vi "Read gesture + average_speed + abs speed - Leap.vi"() -> ()   [LabVIEW 2014]
uses:
  <vilib>/Utility/file.llb/Write To Spreadsheet File (DBL).vi
panel:
  in  "Save":bool
  out "Average Speed":T1(graph)
  out "Absolute speed":T2(graph)
  in  "Acquire":bool
  out "Finger pinch":bool[](array[boolean])
  out "Key tap":string[](array[string])=["Undetected", "Undetected", "Undetected", "Undetected", "Undetected"]
  in  "Key Tap Thresh [degree]":sgl=55.0 caption="Keytap Threshold [degree]"
  out "Wrist Flexion/Extension":string="Undetected"
  in  "Flex-Extension Threshold [degree]":sgl=40.0
  out "Palm State":string="Undetected"
  in  "Stop":bool
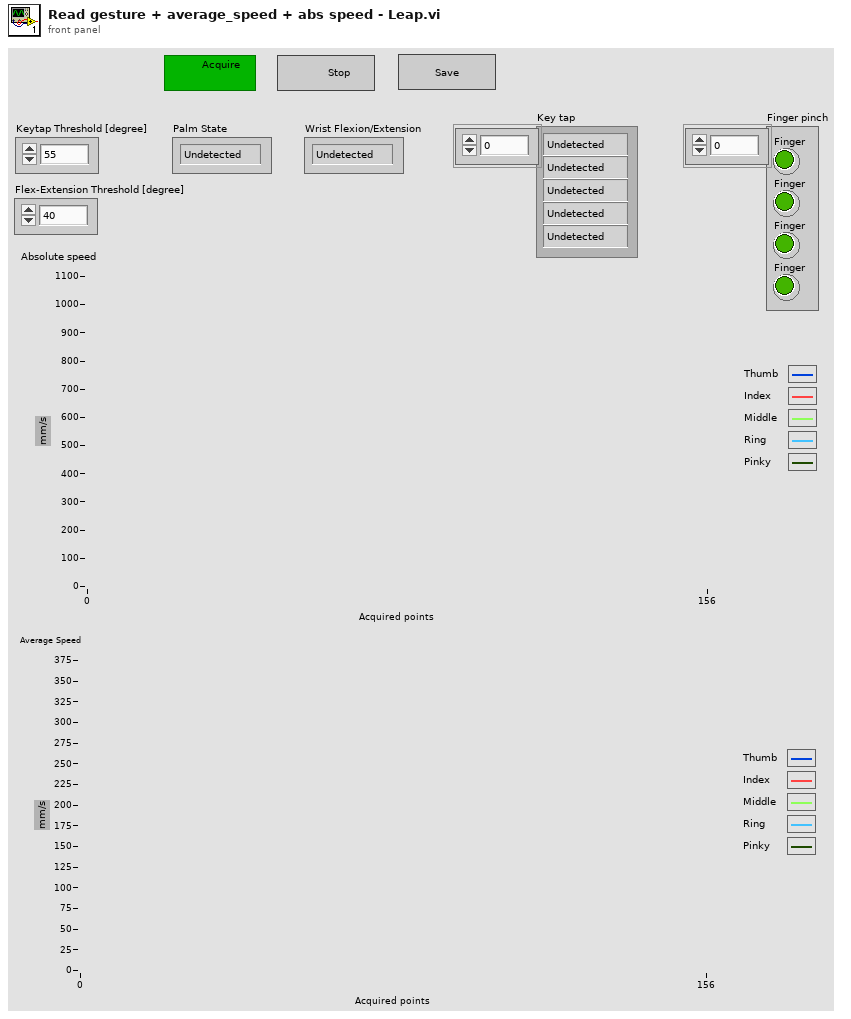
[diagram p1: front panel]
types:
  T1 = cluster{"sqrt(x)":sgl, "sqrt(x)":sgl, "sqrt(x)":sgl, "sqrt(x)":sgl, "sqrt(x)":sgl}
  T2 = cluster{"mean":dbl, "mean":dbl, "mean":dbl, "mean":dbl, "mean":dbl}
  T3 = typedef "Leap Handle.ctl" = cluster{"LeapCSharp":refnum<k24>}
  T4 = cluster{"Numeric":dbl, "Numeric":dbl, "Numeric":dbl, "Numeric":dbl, "Numeric":dbl}
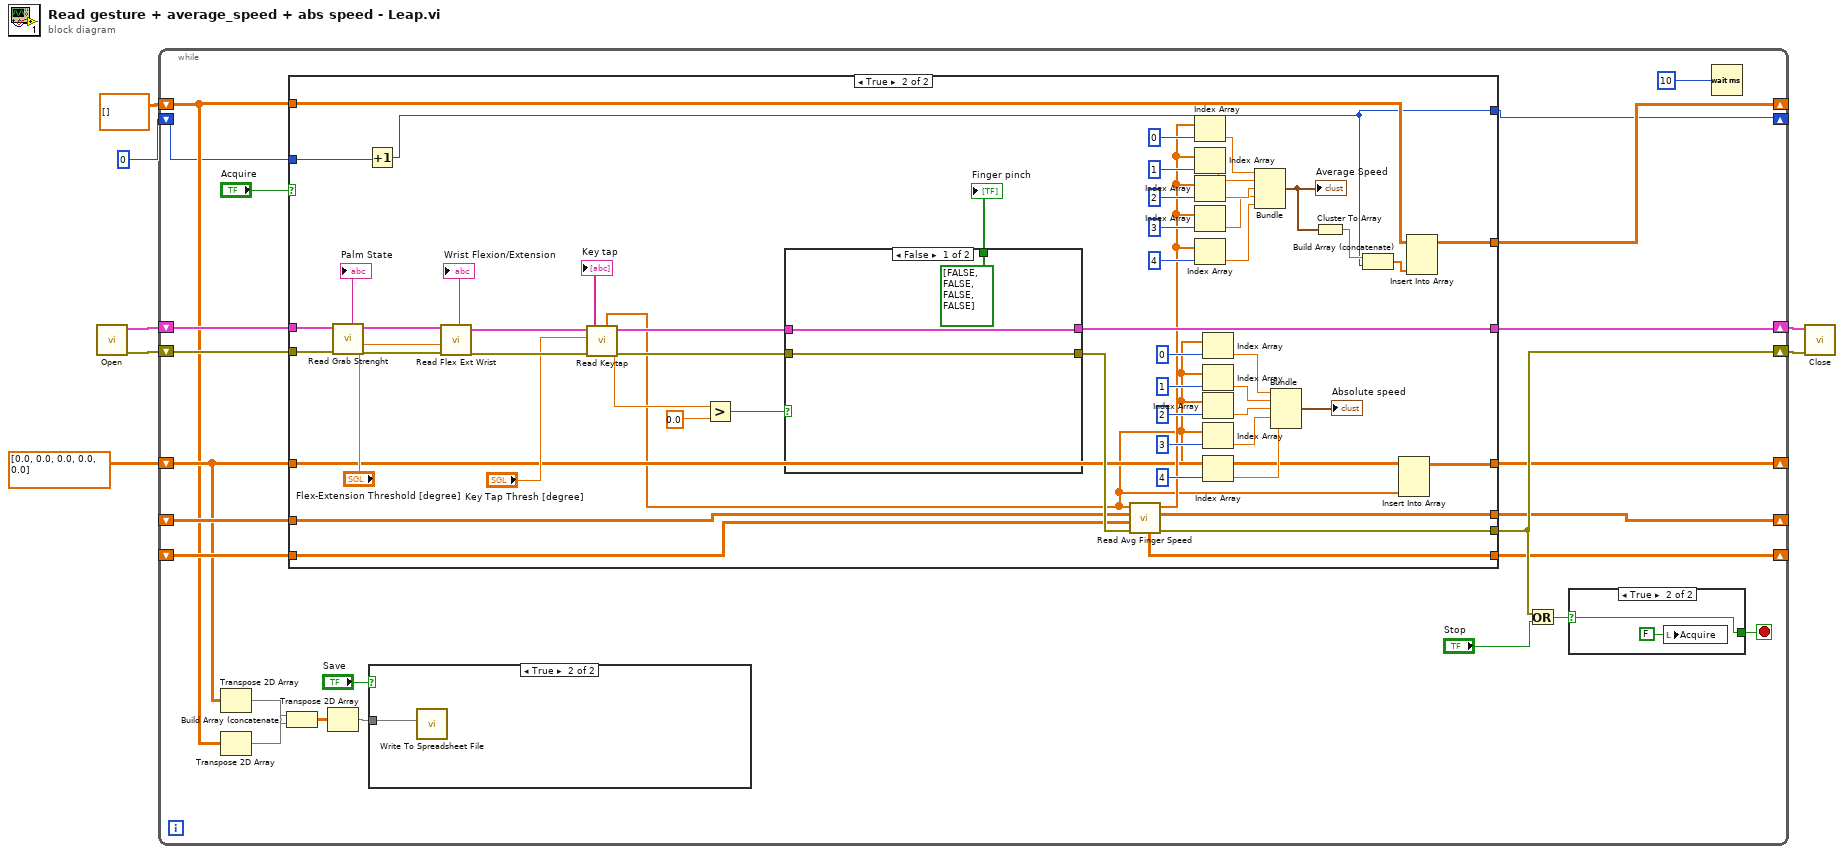
[diagram p0: block diagram]
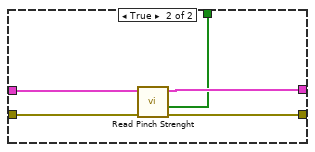
[diagram p5: hidden frame]
diagram:
  n1 = call "Open.vi"() -> ("Error Out"=w6:errorcluster, "Leap Handle"=w7:T3)  [unwired: 10 in]
  n2 = while {
    shift-right: [w27] -> w5
    shift-left: w7 -> [w26]
    shift-right: [w28] -> w4
    shift-left: w6 -> [w29]
    shift-right: [w22] -> _
    shift-left: _ -> [w21]
    shift-right: [w20] -> _
    shift-left: _ -> [w19]
    shift-right: [w18] -> _
    shift-left: sgl[][] [] -> [w14]
    shift-right: [w16] -> _
    shift-left: sgl[][] [[0.0, 0.0, 0.0, 0.0, 0.0]] -> [w15]
    shift-right: [w9] -> _
    shift-left: 0 -> [w8]
    stop <- w23 stop-if-true
    n3 = Transpose 2D Array(2D array=w15) -> (transposed array=w13:sgl[][])
    n4 = Transpose 2D Array(2D array=w14) -> (transposed array=w12:sgl[][])
    n5 = Build Array (concatenate)(w13, w12) -> (w11:sgl[][])
    n6 = case shown="True" "Acquire" {
      tunnel: w29 -> [w41 w98]
      tunnel: [w41 w58] -> w28
      tunnel: [w42 w85] -> w27
      tunnel: w26 -> [w42 w84]
      tunnel: [w38 w60] -> w22
      tunnel: w21 -> [w38 w61]
      tunnel: [w37 w57] -> w20
      tunnel: w19 -> [w37 w56]
      tunnel: [w40 w52] -> w18
      tunnel: w14 -> [w40 w51]
      tunnel: [w39 w49] -> w16
      tunnel: w15 -> [w39 w48]
      tunnel: w8 -> [w36 w46]
      tunnel: [w36 w44] -> w9
      frame False {
      }
      frame True {
        n7 = call "Read Grab Strenght.vi"("Error In"=w98, "Leap Handle In"=w84) -> ("Error Out"=w95:errorcluster, "Leap Handle Out"=w96:T3, "Palm State"=→"Palm State":string)  [unwired: 5 in, 2 out]
        n8 = Increment(x=w46) -> (x+1=w44:i32)
        n9 = call "Read Flex Ext Wrist.vi"("Error In"=w95, "Flex Extension threshold"="Flex-Extension Threshold [degree]", "Leap Handle In"=w96) -> ("Error Out"=w92:errorcluster, "Wrist Flextion/Extension"=→"Wrist Flexion/Extension":string, "Leap Handle Out"=w93:T3)  [unwired: 4 in]
        n10 = call "Read Keytap.vi"("Error In"=w92, "Key Tap Thresh"="Key Tap Thresh [degree]", "Leap Handle In"=w93) -> ("Error Out"=w89:errorcluster, "PinchStrength"=w87:sgl, "Key tap"=→"Key tap":string[], "Leap Handle Out"=w90:T3, "Tip Velocity Module"=w47:dbl[])  [unwired: 3 in]
        n11 = Greater?(x=w87, y=0.0) -> (0:w88:bool)
        n12 = case shown="False" w88 {
          tunnel: w90 -> [w101 w104]
          tunnel: w89 -> [w100 w106]
          tunnel: [w100 w105] -> w62
          tunnel: [w101 w103] -> w85
          tunnel: [bool[] [FALSE, FALSE, FALSE, FALSE] ("Finger pinch") w102] -> w86
          frame False {
          }
          frame True {
            n13 = call "Read Pinch Strenght.vi"("Error In"=w106, "Leap Handle In"=w104) -> ("Error Out"=w105:errorcluster, "Finger pinch"=w102:bool[], "Leap Handle Out"=w103:T3)  [unwired: 6 in, 1 out]
          }
        }
        "Finger pinch" <- w86
        n14 = call "Read Avg Finger Speed.vi"("Tip Velocity Module"=w47, "Array v istantanee  IN"=w61, "Array vel medie IN"=w56, "Error In"=w62) -> ("Array vel medie OUT"=w57:sgl[][], "Velocità medie finali"=w59:sgl[], "Array v istantanee OUT"=w60:sgl[][], "Error Out"=w58:errorcluster)  [unwired: 1 in, 1 out]
        n15 = Index Array(array=w59, index=0) -> (element=w67:sgl)
        n16 = Index Array(array=w59, index=1) -> (element=w66:sgl)
        n17 = Index Array(array=w59, index=2) -> (element=w65:sgl)
        n18 = Index Array(array=w59, index=3) -> (element=w64:sgl)
        n19 = Index Array(array=w59, index=4) -> (element=w63:sgl)
        n20 = Index Array(array=w47, index=0) -> (element=w77:dbl)
        n21 = Index Array(array=w47, index=1) -> (element=w76:dbl)
        n22 = Index Array(array=w47, index=2) -> (element=w75:dbl)
        n23 = Index Array(array=w47, index=3) -> (element=w74:dbl)
        n24 = Index Array(array=w47, index=4) -> (element=w73:dbl)
        n25 = Bundle("sqrt(x)"=w67, "sqrt(x)"=w66, "sqrt(x)"=w65, "sqrt(x)"=w64, "sqrt(x)"=w63) -> (w53:T1)  [unwired: 1 in]
        "Average Speed" <- w53
        n26 = Bundle("Numeric"=w77, "Numeric"=w76, "Numeric"=w75, "Numeric"=w74, "Numeric"=w73) -> (→"Absolute speed":T4)  [unwired: 1 in]
        n27 = Cluster To Array(cluster=w53) -> (array=w45:sgl[])
        n28 = Build Array (concatenate)(w45, w44) -> (w43:sgl[])
        n29 = Insert Into Array(array=w48, new element=w47) -> (w49:sgl[][])  [unwired: 2 in]
        n30 = Insert Into Array(array=w51, new element=w43) -> (w52:sgl[][])  [unwired: 2 in]
      }
    }
    n31 = Transpose 2D Array(2D array=w11) -> (transposed array=w10:sgl[][])
    n32 = case shown="True" "Save" {
      tunnel: w10 -> [_ w32]
      frame False {
      }
      frame True {
        n33 = call-poly <vilib>:"Write To Spreadsheet File.vi"("2D data"=w32) -> ()  [unwired: 7 in, 1 out]
      }
    }
    n34 = Or(x=w28, y="Stop") -> (x .or. y?=w24:bool)
    n35 = case shown="True" w24 {
      selector: w24 -> [w33 w34]
      tunnel: [w33 w34] -> w23
      frame False {
      }
      frame True {
        n36 = local write "Acquire"(FALSE ("Acquire")) -> ()
      }
    }
    n37 = Wait (ms)(milliseconds to wait=u32 10) -> ()  [unwired: 1 out]
  }
  n38 = call "Close.vi"("Error In"=w4, "Leap Handle"=w5) -> ()  [unwired: 9 in, 1 out]
